vi "Excel Input information.vi"(4 "부록용":bool, 6 "문자열":string, 8 "error in":errorcluster caption="에러 입력(에러 없음)", 11 "report in":refnum<class "NI_report.lvclass">) -> (0 "error out":errorcluster caption="에러 출력", 3 "report out":refnum<class "NI_report.lvclass">)   [LabVIEW 2020]
uses:
  <vilib>/Utility/NIReport.llb/NI_report.lvclass
  Variables/Global_Cal Info.vi
  Variables/Global_Cal STD.vi
  <vilib>/Utility/NIReport.llb/Excel/NI_Excel.lvclass
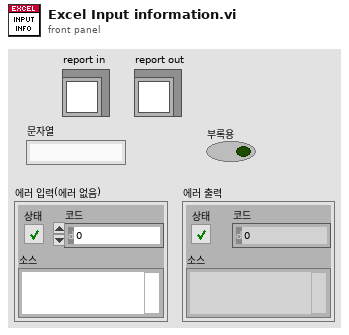
[diagram p1: front panel]
types:
  T1 = typedef "Clst_Cal Info Global.ctl" = cluster{"등록번호":string, "의뢰기관":string, "기기명":string, "제작회사":string, "형식":string, "기기번호":string, "소분류코드":string, "세부분류코드":string, "교정주기":string, "접수번호":string, "교정일자":string, "교정절차서 1":string, "교정절차서 2":string, "교정절차서 3":string, "접수확인자":string, "인증교정자":string, "기술책임자":string, "KOLAS 유무":string, "진행상태":string, "의뢰기관코드":string, "입고형태":string, "영문성적서?":bool, "합불판정?":bool, "부록?":bool, "절차서번호 1":string, "절차서번호 2":string, "절차서번호 3":string, "교정방식":string, "부서명":string}
  T2 = typedef "Clst_Atm Info Global.ctl" = cluster{"교정장소":enum16{"0 : 고정표준실", "1 : 현장교정"}, "최저온도(℃)":string, "최고온도(℃)":string, "최저습도(％ R.H.)":string, "최고습도(％ R.H.)":string, "최저기압(hPa)":string, "최고기압(hPa)":string, "교정실명":string}
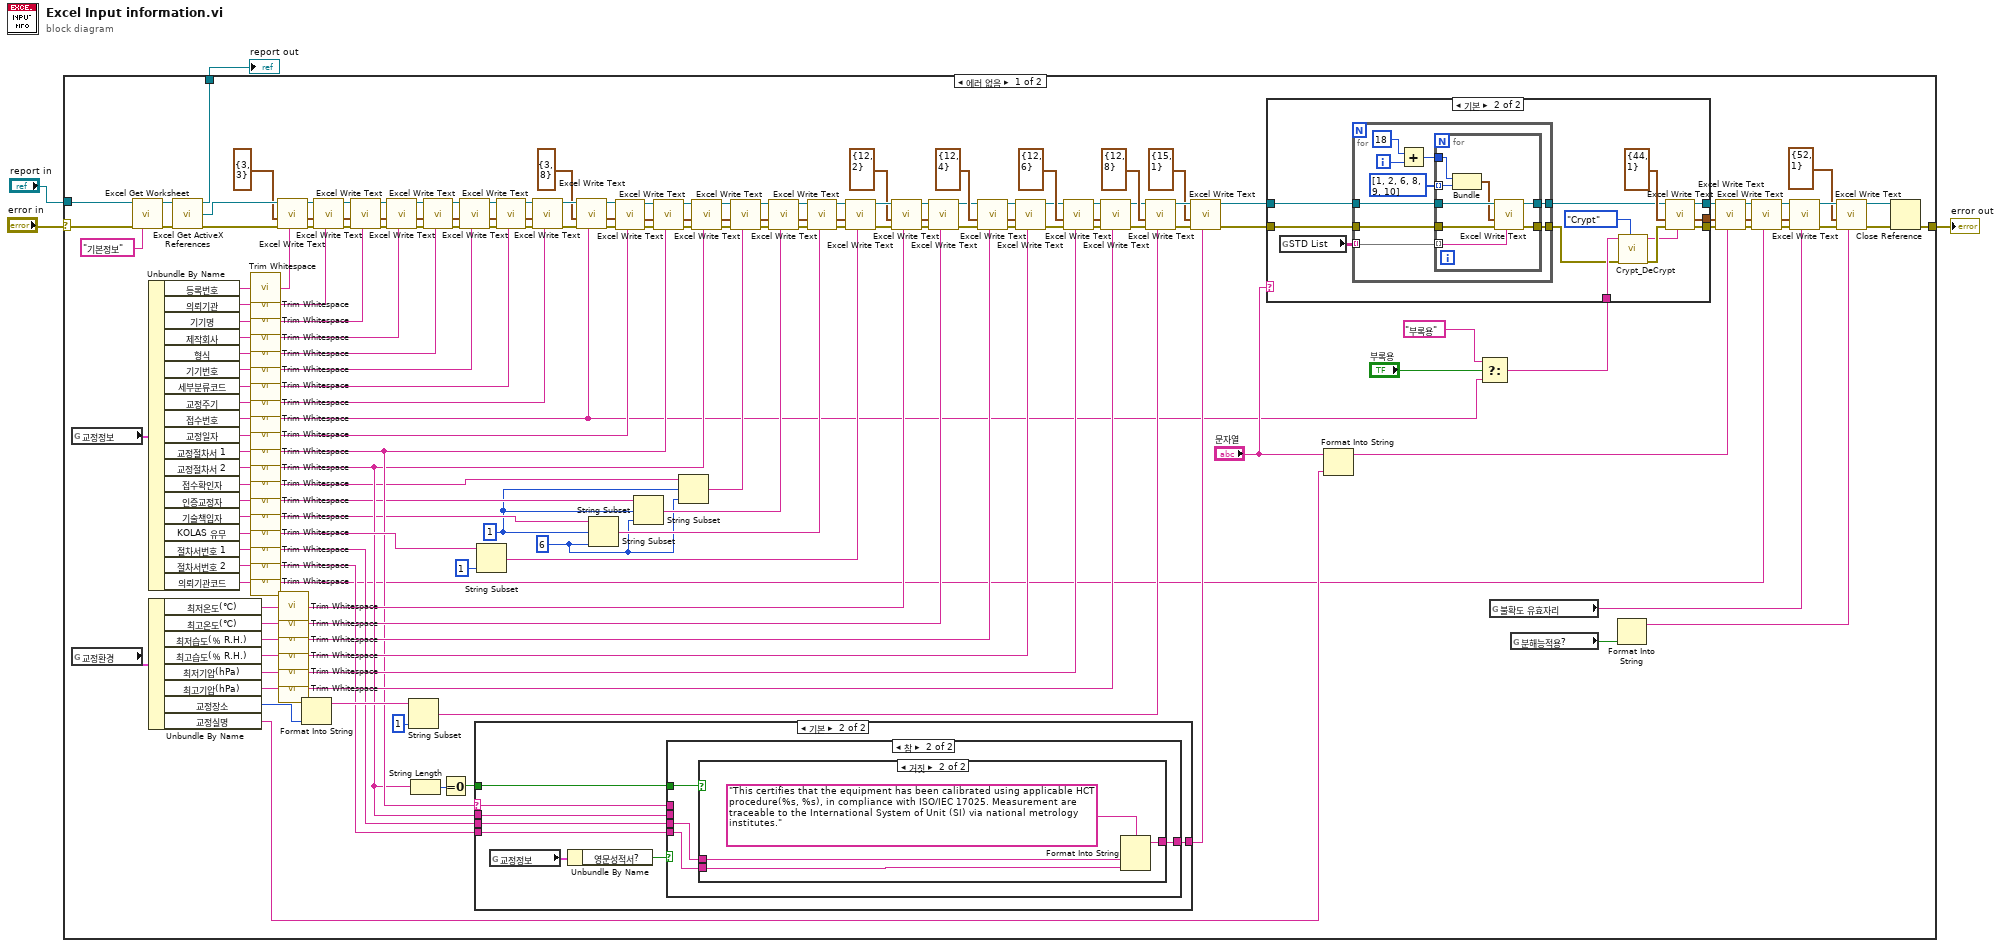
[diagram p0: block diagram]
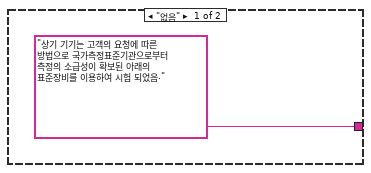
[diagram p2: hidden frame]
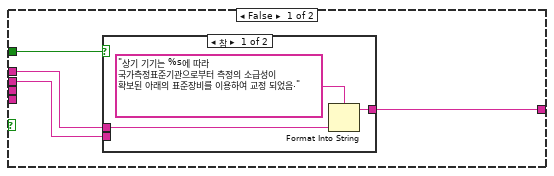
[diagram p3: hidden frame]
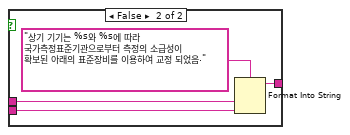
[diagram p4: hidden frame]
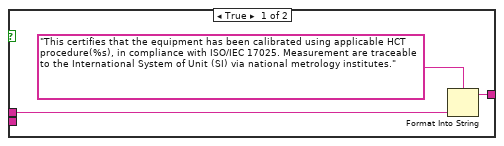
[diagram p5: hidden frame]
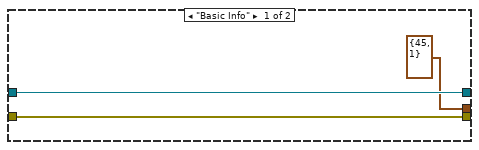
[diagram p6: hidden frame]
diagram:
  n1 = case shown="에러 없음" "error in" {
    selector: "error in" -> [w173 w239]
    tunnel: "report in" -> [w172 w240]
    tunnel: [w169 w240] -> w2
    tunnel: [w55 w239] -> w1
    frame No Error {
      w25 = 1 ("오프셋(0)")
      w26 = 6 ("길이(나머지)")
      n2 = global read "Global_Cal Info.vi" "교정정보"() -> (w165:T1)
      n3 = global read "Global_Cal Info.vi" "교정환경"() -> (w94:T2)
      n4 = call <vilib>:"Excel Get Worksheet.vi"("report in"=w172, "error in (no error)"=w173, "name (\"\")"="기본정보" ("name (\"\")")) -> ("report out"=w171:refnum<class "NI_report.lvclass">, "error out"=w170:errorcluster)  [unwired: 11 in]
      n5 = Unbundle By Name(w165) -> ("등록번호"=w164:string, "의뢰기관"=w160:string, "기기명"=w156:string, "제작회사"=w152:string, "형식"=w148:string, "기기번호"=w144:string, "세부분류코드"=w140:string, "교정주기"=w132:string, "접수번호"=w125:string, "교정일자"=w121:string, "교정절차서 1"=w116:string, "교정절차서 2"=w112:string, "접수확인자"=w107:string, "인증교정자"=w103:string, "기술책임자"=w99:string, "KOLAS 유무"=w95:string, "절차서번호 1"=w40:string, "절차서번호 2"=w38:string, "의뢰기관코드"=w21:string)
      n6 = Unbundle By Name(w94) -> ("최저온도(℃)"=w90:string, "최고온도(℃)"=w85:string, "최저습도(％ R.H.)"=w78:string, "최고습도(％ R.H.)"=w76:string, "최저기압(hPa)"=w69:string, "최고기압(hPa)"=w67:string, "교정장소"=w65:enum16{"0 : 고정표준실", "1 : 현장교정"}, "교정실명"=w46:string)
      n7 = call <vilib>:"Excel Get ActiveX References.vi"("report in"=w171, "error in (no error)"=w170) -> ("report out"=w169:refnum<class "NI_report.lvclass">, "Excel._Worksheet"=w167:refnum<k7>, "error out"=w168:errorcluster)  [unwired: 7 in, 4 out]
      n8 = call <vilib>:"Trim Whitespace.vi"("string"=w164) -> ("trimmed string"=w139:string)  [unwired: 1 in]
      n9 = call <vilib>:"Trim Whitespace.vi"("string"=w160) -> ("trimmed string"=w138:string)  [unwired: 1 in]
      n10 = call <vilib>:"Trim Whitespace.vi"("string"=w156) -> ("trimmed string"=w137:string)  [unwired: 1 in]
      n11 = call <vilib>:"Trim Whitespace.vi"("string"=w152) -> ("trimmed string"=w136:string)  [unwired: 1 in]
      n12 = call <vilib>:"Trim Whitespace.vi"("string"=w148) -> ("trimmed string"=w135:string)  [unwired: 1 in]
      n13 = call <vilib>:"Trim Whitespace.vi"("string"=w144) -> ("trimmed string"=w134:string)  [unwired: 1 in]
      n14 = call <vilib>:"Trim Whitespace.vi"("string"=w140) -> ("trimmed string"=w133:string)  [unwired: 1 in]
      n15 = call <vilib>:"Trim Whitespace.vi"("string"=w132) -> ("trimmed string"=w128:string)  [unwired: 1 in]
      n16 = call <vilib>:"Trim Whitespace.vi"("string"=w125) -> ("trimmed string"=w14:string)  [unwired: 1 in]
      n17 = call <vilib>:"Trim Whitespace.vi"("string"=w121) -> ("trimmed string"=w120:string)  [unwired: 1 in]
      n18 = call <vilib>:"Trim Whitespace.vi"("string"=w116) -> ("trimmed string"=w35:string)  [unwired: 1 in]
      n19 = call <vilib>:"Trim Whitespace.vi"("string"=w112) -> ("trimmed string"=w33:string)  [unwired: 1 in]
      n20 = call <vilib>:"Trim Whitespace.vi"("string"=w107) -> ("trimmed string"=w32:string)  [unwired: 1 in]
      n21 = call <vilib>:"Trim Whitespace.vi"("string"=w103) -> ("trimmed string"=w30:string)  [unwired: 1 in]
      n22 = call <vilib>:"Trim Whitespace.vi"("string"=w99) -> ("trimmed string"=w28:string)  [unwired: 1 in]
      n23 = call <vilib>:"Trim Whitespace.vi"("string"=w95) -> ("trimmed string"=w52:string)  [unwired: 1 in]
      n24 = call <vilib>:"Trim Whitespace.vi"("string"=w40) -> ("trimmed string"=w39:string)  [unwired: 1 in]
      n25 = call <vilib>:"Trim Whitespace.vi"("string"=w38) -> ("trimmed string"=w37:string)  [unwired: 1 in]
      n26 = call <vilib>:"Trim Whitespace.vi"("string"=w21) -> ("trimmed string"=w20:string)  [unwired: 1 in]
      n27 = call "Excel Write Text.vi"("Text"=w139, "error in"=w168, "Address in"=cluster{"Row":i32, "Col":i32} {"Row"=3, "Col"=3} ("Cell in"), "Excel._Worksheet in"=w167) -> ("error out"=w163:errorcluster, "Below Cell"=w162:cluster{"Row":i32, "Column":i32}, "Excel._Worksheet out"=w161:refnum<k7>)  [unwired: 5 in]
      n28 = call <vilib>:"Trim Whitespace.vi"("string"=w90) -> ("trimmed string"=w89:string)  [unwired: 1 in]
      n29 = call <vilib>:"Trim Whitespace.vi"("string"=w85) -> ("trimmed string"=w84:string)  [unwired: 1 in]
      n30 = call <vilib>:"Trim Whitespace.vi"("string"=w78) -> ("trimmed string"=w77:string)  [unwired: 1 in]
      n31 = call <vilib>:"Trim Whitespace.vi"("string"=w76) -> ("trimmed string"=w75:string)  [unwired: 1 in]
      n32 = call <vilib>:"Trim Whitespace.vi"("string"=w69) -> ("trimmed string"=w68:string)  [unwired: 1 in]
      n33 = call <vilib>:"Trim Whitespace.vi"("string"=w67) -> ("trimmed string"=w66:string)  [unwired: 1 in]
      n34 = Format Into String(w65) -> (resulting string=w63:string)  [unwired: 3 in, 1 out]
      n35 = call "Excel Write Text.vi"("Text"=w138, "error in"=w163, "Address in"=w162, "Excel._Worksheet in"=w161) -> ("error out"=w159:errorcluster, "Below Cell"=w158:cluster{"Row":i32, "Column":i32}, "Excel._Worksheet out"=w157:refnum<k7>)  [unwired: 5 in]
      n36 = call "Excel Write Text.vi"("Text"=w137, "error in"=w159, "Address in"=w158, "Excel._Worksheet in"=w157) -> ("error out"=w155:errorcluster, "Below Cell"=w154:cluster{"Row":i32, "Column":i32}, "Excel._Worksheet out"=w153:refnum<k7>)  [unwired: 5 in]
      n37 = call "Excel Write Text.vi"("Text"=w136, "error in"=w155, "Address in"=w154, "Excel._Worksheet in"=w153) -> ("error out"=w151:errorcluster, "Below Cell"=w150:cluster{"Row":i32, "Column":i32}, "Excel._Worksheet out"=w149:refnum<k7>)  [unwired: 5 in]
      n38 = String Subset(string=w63, length (rest)=1 ("길이(나머지)")) -> (substring=w59:string)  [unwired: 1 in]
      n39 = String Length(string=w33) -> (length=w36:i32)
      n40 = call "Excel Write Text.vi"("Text"=w135, "error in"=w151, "Address in"=w150, "Excel._Worksheet in"=w149) -> ("error out"=w147:errorcluster, "Below Cell"=w146:cluster{"Row":i32, "Column":i32}, "Excel._Worksheet out"=w145:refnum<k7>)  [unwired: 5 in]
      n41 = Equal To 0?(x=w36) -> (x = 0?=w34:bool)
      n42 = call "Excel Write Text.vi"("Text"=w134, "error in"=w147, "Address in"=w146, "Excel._Worksheet in"=w145) -> ("error out"=w143:errorcluster, "Below Cell"=w142:cluster{"Row":i32, "Column":i32}, "Excel._Worksheet out"=w141:refnum<k7>)  [unwired: 5 in]
      n43 = case shown="기본" w35 {
        selector: w35 -> [_ w178]
        tunnel: w34 -> [_ w183]
        tunnel: ["상기 기기는 고객의 요청에 따른 방법으로 국가측정표준기관으로부터 측정의 소급성이 확보된 아래의 표준장비를 이용하여 시험 되었음." w182] -> w41
        tunnel: w33 -> [_ w181]
        tunnel: w39 -> [_ w180]
        tunnel: w37 -> [_ w179]
        frame "없음" {
        }
        frame Default {
          n44 = global read "Global_Cal Info.vi" "교정정보"() -> (w177:T1)
          n45 = Unbundle By Name(w177) -> ("영문성적서?"=w176:bool)
          n46 = case shown="참" w176 {
            tunnel: w183 -> [w187 w198]
            tunnel: [w186 w197] -> w182
            tunnel: w178 -> [w185 _]
            tunnel: w181 -> [w184 _]
            tunnel: w180 -> [_ w196]
            tunnel: w179 -> [_ w195]
            frame False {
              n47 = case shown="참" w187 {
                tunnel: w185 -> [w189 w193]
                tunnel: [w188 w191] -> w186
                tunnel: w184 -> [_ w192]
                frame True {
                  n48 = Format Into String(format string="상기 기기는 %s에 따라 국가측정표준기관으로부터 측정의 소급성이 확보된 아래의 표준장비를 이용하여 교정 되었음.", w189) -> (resulting string=w188:string)  [unwired: 2 in, 1 out]
                }
                frame False {
                  n49 = Format Into String(format string="상기 기기는 %s와 %s에 따라 국가측정표준기관으로부터 측정의 소급성이 확보된 아래의 표준장비를 이용하여 교정 되었음.", w193, w192) -> (resulting string=w191:string)  [unwired: 2 in, 1 out]
                }
              }
            }
            frame True {
              n50 = case shown="거짓" w198 {
                tunnel: w196 -> [w200 w204]
                tunnel: [w201 w205] -> w197
                tunnel: w195 -> [_ w203]
                frame True {
                  n51 = Format Into String(format string="This certifies that the equipment has been calibrated using applicable HCT procedure(%s), in compliance with ISO/IEC 17025. Measurement are traceable to the International System of Unit (SI) via national metrology institutes.", w200) -> (resulting string=w201:string)  [unwired: 2 in, 1 out]
                }
                frame False {
                  n52 = Format Into String(format string="This certifies that the equipment has been calibrated using applicable HCT procedure(%s, %s), in compliance with ISO/IEC 17025. Measurement are traceable to the International System of Unit (SI) via national metrology institutes.", w204, w203) -> (resulting string=w205:string)  [unwired: 2 in, 1 out]
                }
              }
            }
          }
        }
      }
      n53 = String Subset(string=w52, length (rest)=1 ("길이(나머지)")) -> (substring=w51:string)  [unwired: 1 in]
      n54 = call "Excel Write Text.vi"("Text"=w133, "error in"=w143, "Address in"=w142, "Excel._Worksheet in"=w141) -> ("error out"=w131:errorcluster, "Below Cell"=w130:cluster{"Row":i32, "Column":i32}, "Excel._Worksheet out"=w129:refnum<k7>)  [unwired: 5 in]
      n55 = call "Excel Write Text.vi"("Text"=w128, "error in"=w131, "Address in"=w130, "Excel._Worksheet in"=w129) -> ("error out"=w127:errorcluster, "Excel._Worksheet out"=w126:refnum<k7>)  [unwired: 5 in, 1 out]
      n56 = call "Excel Write Text.vi"("Text"=w14, "error in"=w127, "Address in"=cluster{"Row":i32, "Col":i32} {"Row"=3, "Col"=8} ("Cell in"), "Excel._Worksheet in"=w126) -> ("error out"=w124:errorcluster, "Below Cell"=w123:cluster{"Row":i32, "Column":i32}, "Excel._Worksheet out"=w122:refnum<k7>)  [unwired: 5 in]
      n57 = String Subset(string=w28, offset (0)=w25, length (rest)=w26) -> (substring=w27:string)
      n58 = call "Excel Write Text.vi"("Text"=w120, "error in"=w124, "Address in"=w123, "Excel._Worksheet in"=w122) -> ("error out"=w119:errorcluster, "Below Cell"=w118:cluster{"Row":i32, "Column":i32}, "Excel._Worksheet out"=w117:refnum<k7>)  [unwired: 5 in]
      n59 = String Subset(string=w30, offset (0)=w25, length (rest)=w26) -> (substring=w29:string)
      n60 = call "Excel Write Text.vi"("Text"=w35, "error in"=w119, "Address in"=w118, "Excel._Worksheet in"=w117) -> ("error out"=w115:errorcluster, "Below Cell"=w114:cluster{"Row":i32, "Column":i32}, "Excel._Worksheet out"=w113:refnum<k7>)  [unwired: 5 in]
      n61 = String Subset(string=w32, offset (0)=w25, length (rest)=w26) -> (substring=w31:string)
      n62 = call "Excel Write Text.vi"("Text"=w33, "error in"=w115, "Address in"=w114, "Excel._Worksheet in"=w113) -> ("error out"=w110:errorcluster, "Below Cell"=w109:cluster{"Row":i32, "Column":i32}, "Excel._Worksheet out"=w108:refnum<k7>)  [unwired: 5 in]
      n63 = call "Excel Write Text.vi"("Text"=w31, "error in"=w110, "Address in"=w109, "Excel._Worksheet in"=w108) -> ("error out"=w106:errorcluster, "Below Cell"=w105:cluster{"Row":i32, "Column":i32}, "Excel._Worksheet out"=w104:refnum<k7>)  [unwired: 5 in]
      n64 = call "Excel Write Text.vi"("Text"=w29, "error in"=w106, "Address in"=w105, "Excel._Worksheet in"=w104) -> ("error out"=w102:errorcluster, "Below Cell"=w101:cluster{"Row":i32, "Column":i32}, "Excel._Worksheet out"=w100:refnum<k7>)  [unwired: 5 in]
      n65 = call "Excel Write Text.vi"("Text"=w27, "error in"=w102, "Address in"=w101, "Excel._Worksheet in"=w100) -> ("error out"=w98:errorcluster, "Below Cell"=w97:cluster{"Row":i32, "Column":i32}, "Excel._Worksheet out"=w96:refnum<k7>)  [unwired: 5 in]
      n66 = call "Excel Write Text.vi"("Text"=w51, "error in"=w98, "Address in"=w97, "Excel._Worksheet in"=w96) -> ("error out"=w93:errorcluster, "Excel._Worksheet out"=w92:refnum<k7>)  [unwired: 5 in, 1 out]
      n67 = call "Excel Write Text.vi"("Text"=w89, "error in"=w93, "Address in"=cluster{"Row":i32, "Col":i32} {"Row"=12, "Col"=2} ("Cell in"), "Excel._Worksheet in"=w92) -> ("error out"=w88:errorcluster, "Below Cell"=w87:cluster{"Row":i32, "Column":i32}, "Excel._Worksheet out"=w86:refnum<k7>)  [unwired: 5 in]
      n68 = call "Excel Write Text.vi"("Text"=w84, "error in"=w88, "Address in"=w87, "Excel._Worksheet in"=w86) -> ("error out"=w82:errorcluster, "Excel._Worksheet out"=w54:refnum<k7>)  [unwired: 5 in, 1 out]
      n69 = call "Excel Write Text.vi"("Text"=w77, "error in"=w82, "Address in"=cluster{"Row":i32, "Col":i32} {"Row"=12, "Col"=4} ("Cell in"), "Excel._Worksheet in"=w54) -> ("error out"=w79:errorcluster, "Below Cell"=w80:cluster{"Row":i32, "Column":i32}, "Excel._Worksheet out"=w83:refnum<k7>)  [unwired: 5 in]
      n70 = call "Excel Write Text.vi"("Text"=w75, "error in"=w79, "Address in"=w80, "Excel._Worksheet in"=w83) -> ("error out"=w71:errorcluster, "Excel._Worksheet out"=w70:refnum<k7>)  [unwired: 5 in, 1 out]
      n71 = call "Excel Write Text.vi"("Text"=w68, "error in"=w71, "Address in"=cluster{"Row":i32, "Col":i32} {"Row"=12, "Col"=6} ("Cell in"), "Excel._Worksheet in"=w70) -> ("error out"=w53:errorcluster, "Below Cell"=w74:cluster{"Row":i32, "Column":i32}, "Excel._Worksheet out"=w72:refnum<k7>)  [unwired: 5 in]
      n72 = call "Excel Write Text.vi"("Text"=w66, "error in"=w53, "Address in"=w74, "Excel._Worksheet in"=w72) -> ("error out"=w61:errorcluster, "Excel._Worksheet out"=w60:refnum<k7>)  [unwired: 5 in, 1 out]
      n73 = call "Excel Write Text.vi"("Text"=w59, "error in"=w61, "Address in"=cluster{"Row":i32, "Col":i32} {"Row"=12, "Col"=8} ("Cell in"), "Excel._Worksheet in"=w60) -> ("error out"=w58:errorcluster, "Excel._Worksheet out"=w57:refnum<k7>)  [unwired: 5 in, 1 out]
      n74 = call "Excel Write Text.vi"("Text"=w41, "error in"=w58, "Address in"=cluster{"Row":i32, "Col":i32} {"Row"=15, "Col"=1} ("Cell in"), "Excel._Worksheet in"=w57) -> ("error out"=w43:errorcluster, "Excel._Worksheet out"=w44:refnum<k7>)  [unwired: 5 in, 1 out]
      n75 = Format Into String(initial string="문자열", w46) -> (resulting string=w45:string)  [unwired: 2 in, 1 out]
      n76 = Select(t="부록용", s="부록용", f=w14) -> (s? t:f=w13:string)
      n77 = case shown="기본" "문자열" {
        tunnel: w13 -> [_ w221]
        tunnel: [w208 w216] -> w49
        tunnel: [w207 w215] -> w48
        tunnel: [cluster{"Row":i32, "Col":i32} {"Row"=45, "Col"=1} ("Cell in") w214] -> w47
        tunnel: w44 -> [w207 w213]
        tunnel: w43 -> [w208 w211]
        frame "Basic Info" {
        }
        frame Default {
          n78 = global read "Global_Cal STD.vi" "STD List"() -> (w209:string[][])
          n79 = for {
            tunnel: w209 -> [w230] mode=indexing
            tunnel: w213 -> [w229]
            tunnel: [w228] -> w210
            tunnel: w211 -> [w226]
            tunnel: [w225] -> w212
            i -> [w223]
            n80 = Add(x=18, y=w223) -> (x+y=w222:i32)
            n81 = for {
              tunnel: w230 -> [w231] mode=indexing
              tunnel: w229 -> [w237]
              tunnel: [w235] -> w228
              tunnel: i32[] [1, 2, 6, 8, 9, 10] -> [w238] mode=indexing
              tunnel: w226 -> [w234]
              tunnel: [w236] -> w225
              tunnel: w222 -> [w232]
              n82 = Bundle(w232, w238) -> (w233:cluster{i32, i32})  [unwired: 1 in]
              n83 = call "Excel Write Text.vi"("Text"=w231, "error in"=w234, "Address in"=w233, "Excel._Worksheet in"=w237) -> ("error out"=w235:errorcluster, "Excel._Worksheet out"=w236:refnum<k7>)  [unwired: 5 in, 1 out]
            }
          }
          n84 = call "Crypt_DeCrypt.vi"("Comm"=enum16{"Crypt", "DeCrypt"}."Crypt", "error in (no error)"=w210, "Texti"=w221) -> ("error out"=w219:errorcluster, "결과"=w217:string)  [unwired: 7 in]
          n85 = call "Excel Write Text.vi"("Text"=w217, "error in"=w219, "Address in"=cluster{"Row":i32, "Col":i32} {"Row"=44, "Col"=1} ("Cell in"), "Excel._Worksheet in"=w212) -> ("error out"=w216:errorcluster, "Below Cell"=w214:cluster{"Row":i32, "Column":i32}, "Excel._Worksheet out"=w215:refnum<k7>)  [unwired: 5 in]
        }
      }
      n86 = global read "Global_Cal Info.vi" "불확도 유효자리"() -> (w16:string)
      n87 = global read "Global_Cal Info.vi" "분해능적용?"() -> (w6:bool)
      n88 = Format Into String(w6) -> (resulting string=w5:string)  [unwired: 3 in, 1 out]
      n89 = call "Excel Write Text.vi"("Text"=w45, "error in"=w49, "Address in"=w47, "Excel._Worksheet in"=w48) -> ("error out"=w24:errorcluster, "Below Cell"=w23:cluster{"Row":i32, "Column":i32}, "Excel._Worksheet out"=w22:refnum<k7>)  [unwired: 5 in]
      n90 = call "Excel Write Text.vi"("Text"=w20, "error in"=w24, "Address in"=w23, "Excel._Worksheet in"=w22) -> ("error out"=w19:errorcluster, "Below Cell"=w18:cluster{"Row":i32, "Column":i32}, "Excel._Worksheet out"=w17:refnum<k7>)  [unwired: 5 in]
      n91 = call "Excel Write Text.vi"("Text"=w16, "error in"=w19, "Address in"=w18, "Excel._Worksheet in"=w17) -> ("error out"=w9:errorcluster, "Excel._Worksheet out"=w11:refnum<k7>)  [unwired: 5 in, 1 out]
      n92 = call "Excel Write Text.vi"("Text"=w5, "error in"=w9, "Address in"=cluster{"Row":i32, "Col":i32} {"Row"=52, "Col"=1} ("Cell in"), "Excel._Worksheet in"=w11) -> ("error out"=w8:errorcluster, "Excel._Worksheet out"=w10:refnum<k7>)  [unwired: 5 in, 1 out]
      n93 = Close Reference(reference=w10, error in (no error)=w8) -> (error out=w55:errorcluster)
    }
    frame Error {
    }
  }
  "report out" <- w2
  "error out" <- w1
